vi "Read Weights.vi"(8 "error in (no error)":errorcluster, 11 "DFT-5 in":refnum<class "DFT5.lvclass">) -> (0 "error out":errorcluster, 2 "Weights":dbl[](array[numeric]), 3 "DFT-5 out":refnum<class "DFT5.lvclass">)   [LabVIEW 2016, in "Exponential Fit Library.lvlib" / "DFT5.lvclass"]
uses:
  DFT5.lvclass
  DFT5.lvclass/DFT5.ctl
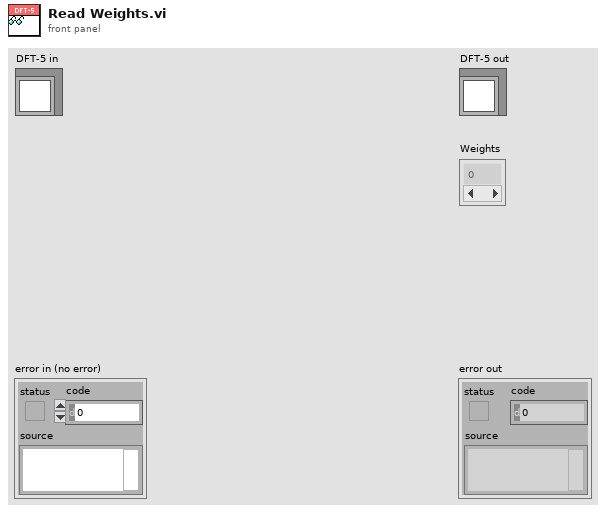
[diagram p1: front panel]
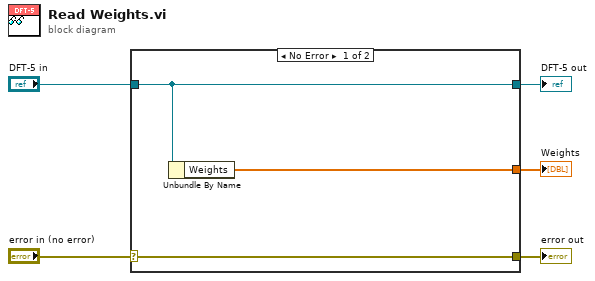
[diagram p0: block diagram]
diagram:
  n1 = case shown="No Error" "error in (no error)" {
    selector: "error in (no error)" -> [w8 w9]
    tunnel: [w8 w9] -> w4
    tunnel: [w7 w10] -> w2
    tunnel: "DFT-5 in" -> [w7 w10]
    tunnel: [w6 _] -> w1
    frame No Error {
      n2 = Unbundle By Name(w7) -> ("Weights"=w6:dbl[])
    }
    frame Error {
    }
  }
  "error out" <- w4
  "DFT-5 out" <- w2
  "Weights" <- w1
